vi "Main UI Initial Staates.vi"(10 "UI References":T1) -> ()   [LabVIEW 2019]
uses:
  TypeDef/UI References.ctl
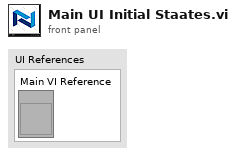
[diagram p1: front panel]
types:
  T1 = typedef "UI References.ctl" = cluster{"Main VI Reference":refnum<vi>}
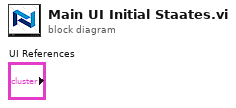
[diagram p0: block diagram]
diagram:
